vi "Set Button From Vi.vi"(0 "Display State In":T3={"Buttons Displayed"=0, "Button States"=[], "Button Size"=0, "Button Style"=enum."Classic", "Active Button"=0, "Force Regen?"=FALSE, "Tip String Ref"=refnum}, 1 "Button Index":i32, 2 "State":T2, 3 "Type":T1, 5 "VI Refnum":refnum<vi>, 9 "Container State":T5, 11 "error in (no error)":errorcluster) -> (4 "Display State Out":T3={"Buttons Displayed"=0, "Button States"=[], "Button Size"=0, "Button Style"=enum."Classic", "Active Button"=0, "Force Regen?"=FALSE, "Tip String Ref"=refnum}, 15 "error out":errorcluster)   [LabVIEW 2012, in "Toolbar.xctl"]
uses:
  Toolbar.xctl
  <vilib>/_xctls/Container State.ctl
  Toolbar State.ctl
  Button_Class/Button.lvclass
  Button_Class/Type Defs/Button Style.ctl
  Button_Class/Type Defs/Button Status.ctl
  Button_Class/Type Defs/Button Type.ctl
  <userlib>/_OpenG.lib/file/file.llb/Strip Path Extension - String__ogtk.vi
  <vilib>/_xctls/XControlSupport.lvlib
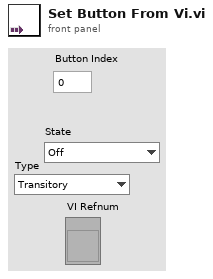
[diagram p1: front panel]
types:
  T1 = typedef "Button.lvclass/Button Type.ctl" = enum16{"Transitory", "Latching"}
  T2 = typedef "Button.lvclass/Button Status.ctl" = enum16{"Off", "Hover", "On", "Disabled"}
  T3 = typedef "Toolbar.xctl/Toolbar State.ctl" = cluster{"Buttons Displayed":i32, "Button States":refnum<class "Button.lvclass">[], "Button Size":i32, "Button Style":T4, "Active Button":i32, "Force Regen?":bool, "Tip String Ref":refnum<vi>}
  T4 = typedef "Button.lvclass/Button Style.ctl" = enum16{"System", "Modern", "Classic", "Rounded", "Silver", "Ni Theme", "Metallic"}
  T5 = typedef "XControlSupport.lvlib/Container State.ctl" = cluster{"Indicator?":bool, "Run Mode?":bool, " Refnum":refnum<vi>}
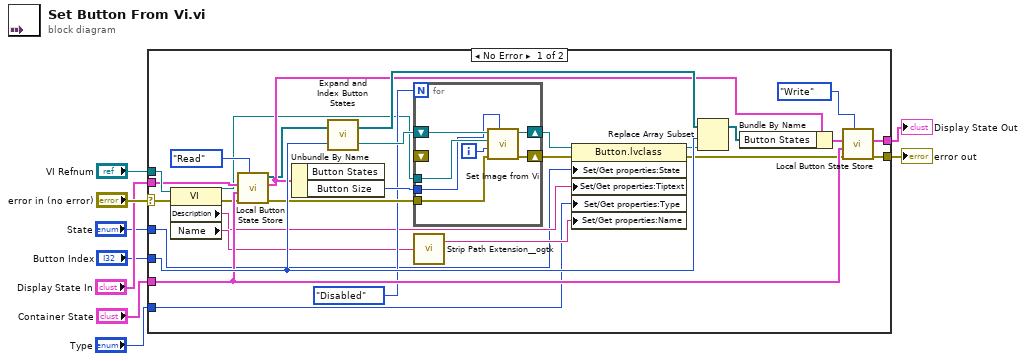
[diagram p0: block diagram]
diagram:
  n1 = case shown="No Error" "error in (no error)" {
    selector: "error in (no error)" -> [w11 w46]
    tunnel: "Display State In" -> [w25 w47]
    tunnel: [w26 w47] -> w4
    tunnel: [w28 w46] -> w3
    tunnel: "Button Index" -> [w37 _]
    tunnel: "State" -> [w12 _]
    tunnel: "VI Refnum" -> [w34 _]
    tunnel: "Container State" -> [w22 _]
    tunnel: "Type" -> [w13 _]
    frame No Error {
      n2 = property class="VI"(reference=w34, error in=w11) -> (reference out=w20:refnum<vi>, error out=w10:errorcluster, "Description"=w14:string, "Name"=w16:string)
      n3 = call "Local Button State Store.vi"("Operation"=enum16{"Read", "Write"}."Read", "error in (no error)"=w10, "Container State"=w22, "Display State In"=w25) -> ("error out"=w32:errorcluster, "Display State Out"=w24:T3, "Button States"=w23:refnum<class "Button.lvclass">[])  [unwired: 5 out]
      n4 = Unbundle By Name(w24) -> ("Button Size"=w33:i32)  [unwired: 1 out]
      n5 = call "Expand and Index Button States.vi"("Button Index"=w37, "Button States"=w23) -> ("Button.lvclass"=w36:refnum<class "Button.lvclass">, "Button States Out"=w38:refnum<class "Button.lvclass">[])
      n6 = for {
        N: Button_Status."Disabled" ("State") -> [_]
        tunnel: w20 -> [w43]
        tunnel: w33 -> [w42]
        tunnel: w32 -> [w41]
        shift-right: [w44] -> w35
        shift-left: w36 -> [w45]
        shift-right: [w40] -> w18
        shift-left: _ -> [_]
        i -> [w39]
        n7 = call-dynamic "Set Image from Vi.vi"("Button Size"=w42, "error in (no error)"=w41, "State"=w39, "VI Refnum"=w43, "Button in"=w45) -> ("error out"=w40:errorcluster, "Button out"=w44:refnum<class "Button.lvclass">)  [unwired: 1 in, 4 out]
      }
      n8 = call-poly <userlib>:"Strip Path Extension__ogtk.vi"("path"=w16) -> ("root"=w15:string)  [unwired: 1 out]
      n9 = property class="Button.lvclass"(reference=w35, error in=w18, "Set/Get properties:State"=w12, "Set/Get properties:Tiptext"=w14, "Set/Get properties:Type"=w13, "Set/Get properties:Name"=w15) -> (reference out=w19:refnum<class "Button.lvclass">, error out=w17:errorcluster)
      n10 = Replace Array Subset(array=w38, new element=w19, index=w37) -> (w30:refnum<class "Button.lvclass">[])
      n11 = Bundle By Name(cluster=w24, "Button States"=w30) -> (w27:T3)
      n12 = call "Local Button State Store.vi"("Operation"=enum16{"Read", "Write"}."Write", "error in (no error)"=w17, "Container State"=w22, "Display State In"=w27) -> ("error out"=w28:errorcluster, "Display State Out"=w26:T3)  [unwired: 1 in, 5 out]
    }
    frame Error {
    }
  }
  "Display State Out" <- w4
  "error out" <- w3
